vi "Get Assertion Result.vi"(8 "error in (no error)":errorcluster, 11 "Test VIs":T4) -> (0 "error out":errorcluster, 2 "Results":T1[](array[typedef]), 3 "First Result":T1={"Name"="", "Description"="", "Status"=enum."Passed", "Result Type"=enum."Test Suite", "Execution Time"=0.0, "Data"={"Expected"=variant, "Actual"=variant, "Delta"=variant}})   [LabVIEW 2020, in "Compare Assertion Test.lvclass"]
uses:
  Compare Assertion Test.lvclass
  Comparison Test Double/Test Methods.ctl
  source/Core/Result/Result.ctl
  source/Core/Result/Status.ctl
  source/Core/Result/Type.ctl
  Comparison Test Double/Comparison Test Double.lvclass
  C:/git/astemes-lunit/source/Core/LUnit Test Case/LUnit Test Case.lvclass
  source/LUnit Test Case.lvclass/LUnit Test Case.ctl
  <vilib>/Utility/LVClass/Get LV Class Name.vi
  source/LUnit Test Case.lvclass
  source/Core/Result/Result.lvlib
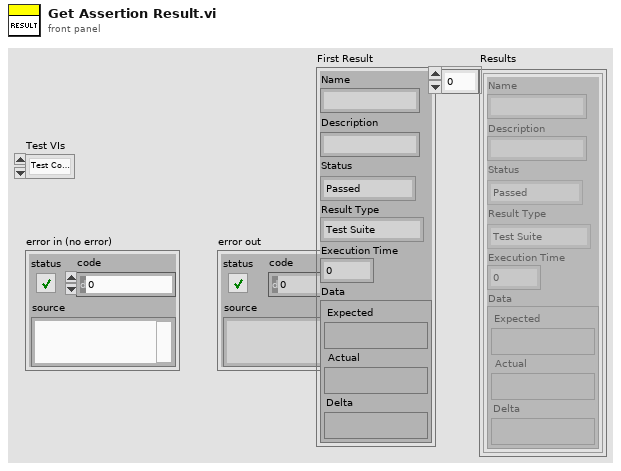
[diagram p1: front panel]
types:
  T1 = typedef "Result.lvlib/Result.ctl" = cluster{"Name":string, "Description":string, "Status":T2, "Result Type":T3, "Execution Time":dbl, "Data":cluster{"Expected":variant, "Actual":variant, "Delta":variant}}
  T2 = typedef "Result.lvlib/Status.ctl" = enum16{"", "Passed", "Failed", "Error", "Skipped", "Setup Error", "Broken", "Teardown Error"}
  T3 = typedef "Result.lvlib/Type.ctl" = enum16{"Test Case", "Test Suite", "Test Run", "Pass", "Fail", "Skip", "Pass if", "Fail if", "Pass if Error", "Fail if Error", "Pass if Equal", "Fail if Equal"}
  T4 = typedef "Comparison Test Double.lvclass/Test Methods.ctl" = enum16{"Test Compare Equal Enums.vi", "Test Compare Unequal Enums.vi", "Test Compare Equal Strings.vi", "Test Compare Unequal Type Deffed Enums.vi", "Test Compare Equal 8bit Enums.vi", "Test Compare Equal 1el String Arrays.vi", "Test Compare Fail if Equal 1el String Arrays.vi", "Test Compare Array with Tolerance.vi", "Test Compare Equal Strings one as Variant.vi", "Test Compare Equal Strings Other as Variant.vi", "Test Compare Equal Variants.vi", "Test Compare Equal Clusters.vi", "Test Compare Equal Nested Clusters.vi", "Test Compare Equal Arrays of Clusters.vi", "Test Compare Empty Array.vi", "Test Compare Equal Strings one Typedef.vi", "Test Compare Equal NaNs.vi"}
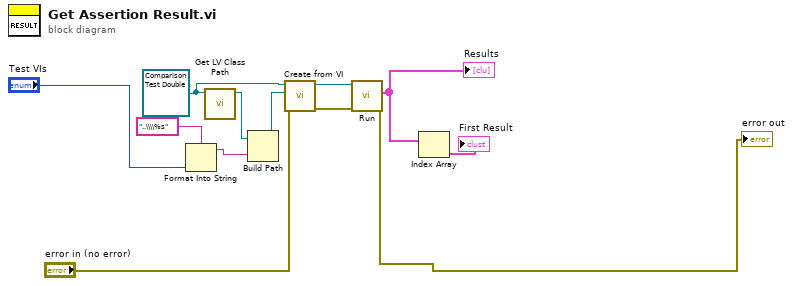
[diagram p0: block diagram]
diagram:
  w4 = refnum<class "Comparison Test Double.lvclass"> refnum ("Comparison Test Double.lvclass")
  n1 = Format Into String(format string="..\\\\%s", "Test VIs") -> (resulting string=w9:string)  [unwired: 2 in, 1 out]
  n2 = call <vilib>:"Get LV Class Path.vi"("object"=w4) -> ("class path"=w6:path)  [unwired: 9 in, 1 out]
  n3 = Build Path(base path=w6, name or relative path=w9) -> (appended path=w3:path)
  n4 = call "Create from VI.vi"("error in (no error)"="error in (no error)", "Test Method VI Path"=w3, "LUnit Test Case In"=w4) -> ("error out"=w1:errorcluster, "LUnit Test Case Out"=w11:refnum<class "Comparison Test Double.lvclass">)  [unwired: 7 in]
  n5 = call-dynamic "Run.vi"("error in (no error)"=w1, "LUnit Test Case In"=w11) -> ("error out"=→"error out":errorcluster, "Results"=w12:T1[])  [unwired: 6 in, 2 out]
  "Results" <- w12
  n6 = Index Array(array=w12) -> (element=→"First Result":T1)  [unwired: 1 in]
